vi "EmptyLabels.vi"(8 "?":T1={"Numeric"=1234.0, "Enum"=enum."Two", "Ring"=10, {"Enum 2"=enum."Two - 2", "Ring 2"=10}} {"?"."Ring 2" items=["Four - 4"=4, "Seven - 7"=7, "Ten - 10"=10, "Twenty - 20"=20]; "Ring" items=["Four"=4, "Seven"=7, "Ten"=10, "Twenty"=20]}, 9 "Cluster 3":T2={"Numeric"=1234.0, enum."Two", 10, {"Enum"=enum."Two - 2", "Ring"=10}} {"?"."Ring" items=["Four - 4"=4, "Seven - 7"=7, "Ten - 10"=10, "Twenty - 20"=20]; "?" items=["Four"=4, "Seven"=7, "Ten"=10, "Twenty"=20]}, 10 "Cluster 2":T3={"Numeric"=1234.0, enum."Two", 10, {enum."Two - 2", 10}} {"?"."?" items=["Four - 4"=4, "Seven - 7"=7, "Ten - 10"=10, "Twenty - 20"=20]; "?" items=["Four"=4, "Seven"=7, "Ten"=10, "Twenty"=20]}, 11 "Cluster":T4={"Numeric"=1234.0, enum."Two", 10, "Cluster"={enum."Two - 2", 10}} {"Cluster"."?" items=["Four - 4"=4, "Seven - 7"=7, "Ten - 10"=10, "Twenty - 20"=20]; "?" items=["Four"=4, "Seven"=7, "Ten"=10, "Twenty"=20]}) -> ()   [LabVIEW 2011]
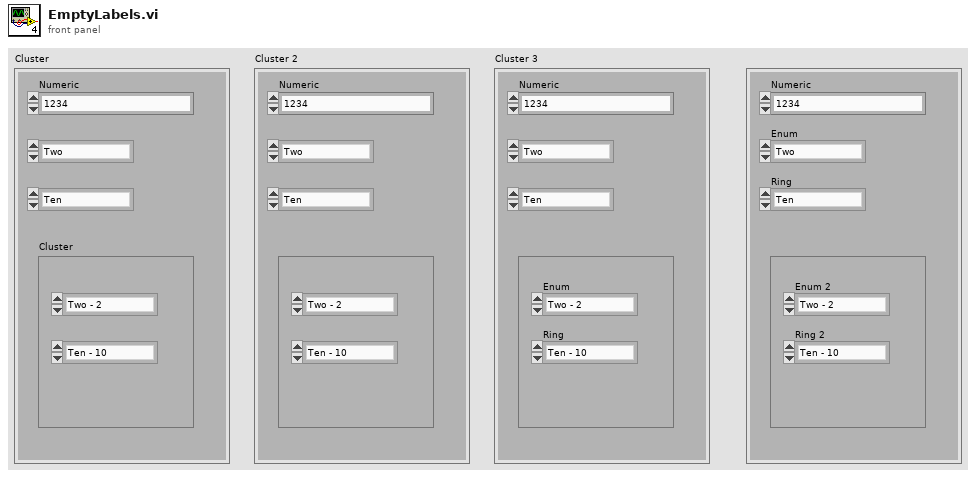
[diagram p1: front panel]
types:
  T1 = cluster{"Numeric":dbl, "Enum":enum16{"Zero", "One", "Two", "Three"}, "Ring":u16, cluster{"Enum 2":enum16{"Zero - 0", "One - 1", "Two - 2", "Three - 3"}, "Ring 2":u16}}
  T2 = cluster{"Numeric":dbl, enum16{"Zero", "One", "Two", "Three"}, u16, cluster{"Enum":enum16{"Zero - 0", "One - 1", "Two - 2", "Three - 3"}, "Ring":u16}}
  T3 = cluster{"Numeric":dbl, enum16{"Zero", "One", "Two", "Three"}, u16, cluster{enum16{"Zero - 0", "One - 1", "Two - 2", "Three - 3"}, u16}}
  T4 = cluster{"Numeric":dbl, enum16{"Zero", "One", "Two", "Three"}, u16, "Cluster":cluster{enum16{"Zero - 0", "One - 1", "Two - 2", "Three - 3"}, u16}}
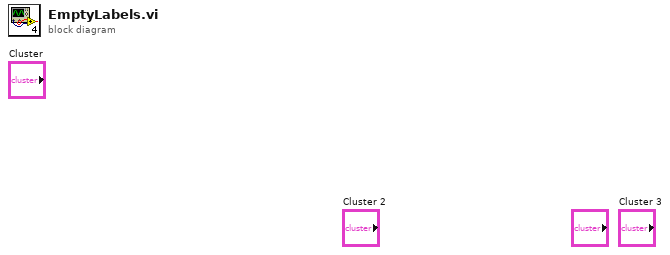
[diagram p0: block diagram]
diagram:
